vi "Init.vi"(5 "Bus In":refnum<class "Bus.lvclass">, 7 "Cluster":T1, 8 "error in (no error)":errorcluster, 9 "Init or Array":bool, 10 "Array":dbl[](array[numeric]), 11 "No Out in":refnum<class "No Output.lvclass">) -> (0 "error out":errorcluster, 2 "Bus Out":refnum<class "Bus.lvclass">, 3 "No Out out":refnum<class "No Output.lvclass">)   [LabVIEW 2024, in "No Output.lvclass"]
uses:
  No Output.lvclass
  Scaling/Scaling.lvclass
  Bus/Bus.lvclass
  No Output.lvclass/No Output.ctl
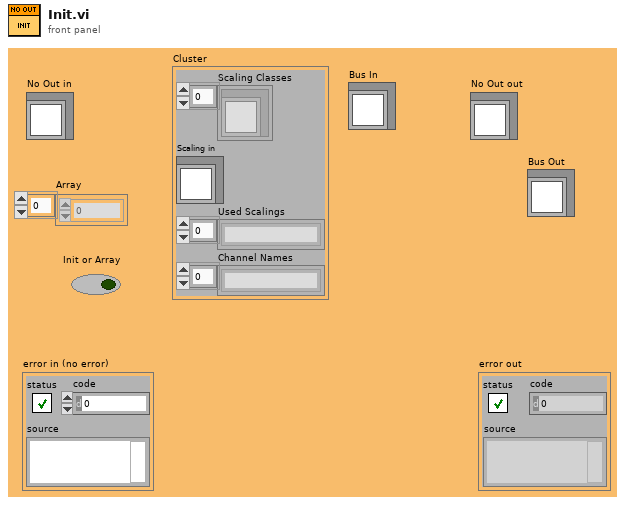
[diagram p1: front panel]
types:
  T1 = cluster{"Scaling Classes":refnum<class "Scaling.lvclass">[], "Scaling in":refnum<class "Scaling.lvclass">, "Used Scalings":string[], "Channel Names":string[]}
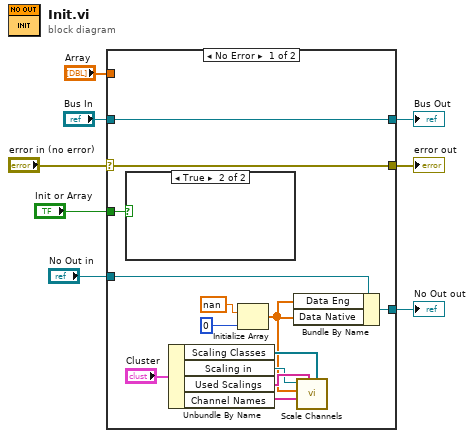
[diagram p0: block diagram]
diagram:
  n1 = case shown="No Error" "error in (no error)" {
    selector: "error in (no error)" -> [w21 w23]
    tunnel: [w21 w23] -> w7
    tunnel: [w20 w24] -> w5
    tunnel: "No Out in" -> [w19 w24]
    tunnel: "Init or Array" -> [w16 _]
    tunnel: "Array" -> [_ _]
    tunnel: "Bus In" -> [w9 w22]
    tunnel: [w9 w22] -> w1
    frame No Error {
      n2 = case shown="True" w16 {
        frame False {
        }
        frame True {
        }
      }
      n3 = Unbundle By Name("Cluster") -> ("Scaling Classes"=w12:refnum<class "Scaling.lvclass">[], "Scaling in"=w13:refnum<class "Scaling.lvclass">, "Used Scalings"=w14:string[], "Channel Names"=w15:string[])
      n4 = Initialize Array(nan ("element"), 0 ("dimension size")) -> (w10:dbl[])
      n5 = Bundle By Name(cluster=w19, "Data Eng"=w10, "Data Native"=w10) -> (w20:refnum<class "No Output.lvclass">)
      n6 = call "Scale Channels.vi"("Scaling Classes"=w12, "Used Scalings"=w14, "Channel Names"=w15, "Values In"=w10, "Scaling in"=w13) -> ()  [unwired: 4 in, 3 out]
    }
    frame Error {
    }
  }
  "error out" <- w7
  "No Out out" <- w5
  "Bus Out" <- w1
